vi "SP Align N Complex Waveforms (Linear Interpolation).vi"(4 "Interpolation":bool=TRUE, 5 "Exported Interval":enum16{"Common", "Global"}(ring), 7 "Open Interval? (T)":bool=TRUE, 8 "error in (no error)":errorcluster, 11 "Waveforms In":waveform(cdb)[](array[waveform])) -> (0 "error out":errorcluster, 3 "Aligned Waveforms In":waveform(cdb)[](array[waveform]))   [LabVIEW 2011]
panel:
  in  "Waveform":waveform(cdb)
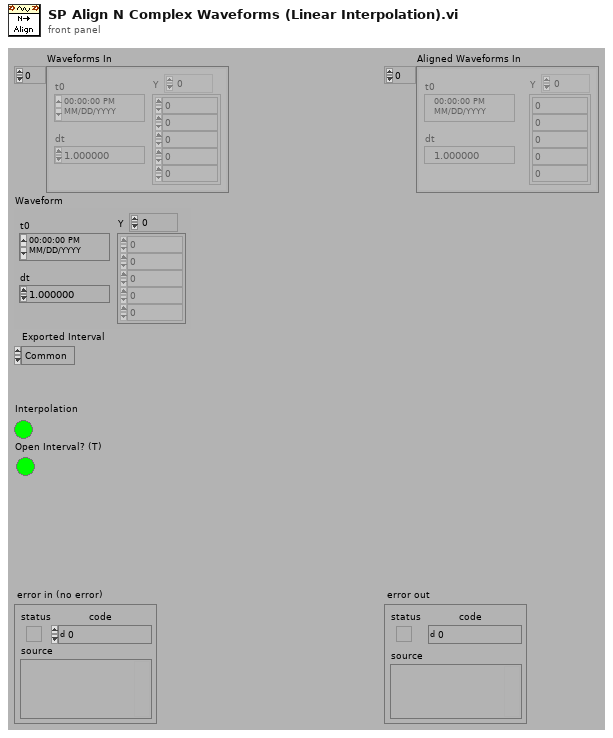
[diagram p1: front panel]
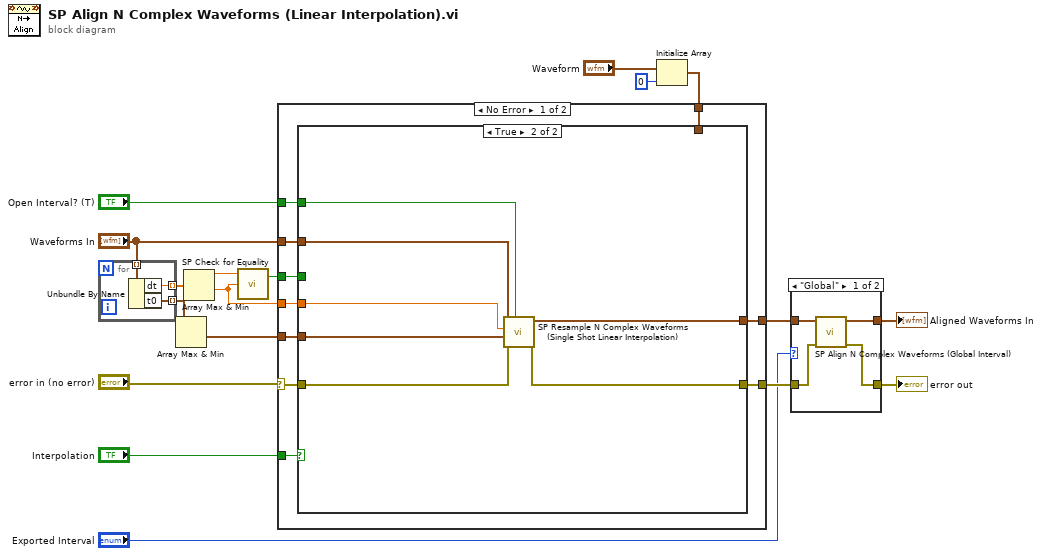
[diagram p0: block diagram]
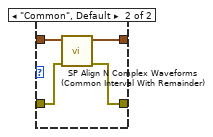
[diagram p2: hidden frame]
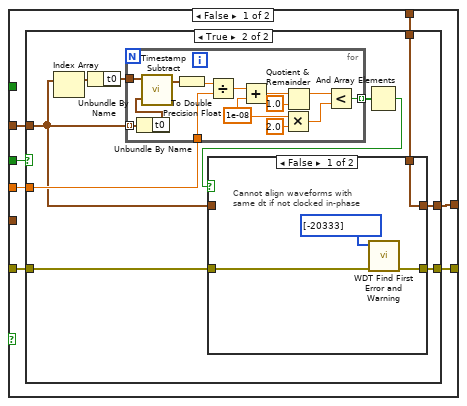
[diagram p3: hidden frame]
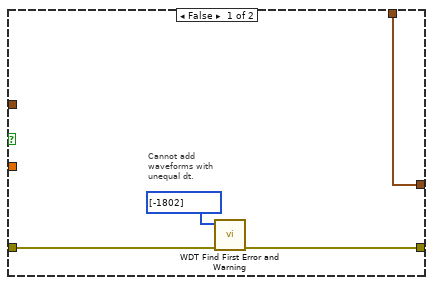
[diagram p4: hidden frame]
diagram:
  n1 = for {
    tunnel: "Waveforms In" -> [w21] mode=indexing
    tunnel: [w20] -> w18 mode=indexing
    tunnel: [w19] -> w2 mode=indexing
    n2 = Unbundle By Name(w21) -> ("dt"=w20:dbl, "t0"=w19:timestamp)
  }
  n3 = Array Max & Min(array=w2) -> (min value=w1:timestamp)  [unwired: 3 out]
  n4 = Array Max & Min(array=w18) -> (max value=w5:dbl, min value=w4:dbl)  [unwired: 2 out]
  n5 = call "SP Check for Equality.vi"("n2"=w4, "n1"=w5) -> ("equal?"=w3:bool)  [unwired: 1 in, 1 out]
  n6 = Initialize Array("Waveform", 0 ("dimension size")) -> (w7:waveform(cdb)[])
  n7 = case shown="No Error" "error in (no error)" {
    selector: "error in (no error)" -> [w30 w81]
    tunnel: [w29 w81] -> w14
    tunnel: w7 -> [w31 w80]
    tunnel: [w28 w80] -> w15
    tunnel: "Interpolation" -> [w27 _]
    tunnel: "Open Interval? (T)" -> [w26 _]
    tunnel: w4 -> [w25 _]
    tunnel: "Waveforms In" -> [w24 _]
    tunnel: w3 -> [w23 _]
    tunnel: w1 -> [w22 _]
    frame No Error {
      n8 = case shown="True" w27 {
        tunnel: w31 -> [w38 _]
        tunnel: w30 -> [w37 w78]
        tunnel: [w36 w79] -> w29
        tunnel: [w35 w74] -> w28
        tunnel: w26 -> [_ w77]
        tunnel: w25 -> [w33 w76]
        tunnel: w24 -> [w32 w75]
        tunnel: w23 -> [w34 _]
        tunnel: w22 -> [_ w73]
        frame False {
          n9 = case shown="True" w34 {
            tunnel: w38 -> [w39 w50]
            tunnel: w37 -> [w42 w52]
            tunnel: [w41 w51] -> w36
            tunnel: [w39 w49] -> w35
            tunnel: w33 -> [_ w48]
            tunnel: w32 -> [_ w44]
            frame False {
              # "Cannot add\nwaveforms with\nunequal dt."
              n10 = call <vilib>:"WDT Find First Error and Warning.vi"("error in (no error)"=w42, "Error Codes"=i32[] [-1802]) -> ("error out"=w41:errorcluster)  [unwired: 1 in, 4 out]
            }
            frame True {
              n11 = Index Array(array=w44) -> (element=w47:waveform(cdb))  [unwired: 1 in]
              n12 = Unbundle By Name(w47) -> ("t0"=w43:timestamp)
              n13 = for {
                tunnel: w43 -> [w56]
                tunnel: w48 -> [w60]
                tunnel: [w64] -> w46 mode=indexing
                tunnel: w44 -> [w59] mode=indexing
                w57 = 1e-08
                n14 = Unbundle By Name(w59) -> ("t0"=w55:timestamp)
                n15 = call <vilib>:"Timestamp Subtract.vi"("y"=w55, "x"=w56) -> ("x - y"=w54:timestamp)
                n16 = To Double Precision Float(number=w54) -> (double precision float=w53:dbl)
                n17 = Divide(x=w53, y=w60) -> (x/y=w58:dbl)
                n18 = Add(x=w58, y=w57) -> (x+y=w63:dbl)
                n19 = Multiply(x=w57, y=2.0) -> (x*y=w61:dbl)
                n20 = Quotient & Remainder(x=w63, y=1.0) -> (x-y*floor(x/y)=w65:dbl)  [unwired: 1 out]
                n21 = Less?(x=w65, y=w61) -> (x < y?=w64:bool)
              }
              n22 = And Array Elements(Boolean array=w46) -> (logical AND=w45:bool)
              n23 = case shown="False" w45 {
                tunnel: [w68 w71] -> w51
                tunnel: w52 -> [w67 w71]
                tunnel: w50 -> [w70 _]
                tunnel: w44 -> [_ w72]
                tunnel: [w70 w72] -> w49
                frame False {
                  # "Cannot align waveforms with\nsame dt if not clocked in-phase"
                  n24 = call <vilib>:"WDT Find First Error and Warning.vi"("error in (no error)"=w67, "Error Codes"=i32[] [-20333]) -> ("error out"=w68:errorcluster)  [unwired: 1 in, 4 out]
                }
                frame True {
                }
              }
            }
          }
        }
        frame True {
          n25 = call "SP Resample N Complex Waveforms (Single Shot Linear Interpolation).vi"("open interval? (T)"=w77, "error in (no error)"=w78, "t0"=w73, "dt"=w76, "waveforms in"=w75) -> ("error out"=w79:errorcluster, "resampled waveforms out"=w74:waveform(cdb)[])  [unwired: 5 out]
        }
      }
    }
    frame Error {
      # "An empty waveform is \nwritten out"
      # "Incoming Error"
    }
  }
  n26 = case shown="\"Global\"" "Exported Interval" {
    tunnel: w15 -> [w83 w86]
    tunnel: [w85 w89] -> w13
    tunnel: w14 -> [w84 w88]
    tunnel: [w82 w87] -> w6
    frame "Global" {
      n27 = call "SP Align N Complex Waveforms (Global Interval).vi"("error in"=w84, "waveforms in"=w83) -> ("error out"=w85:errorcluster, "waveforms out"=w82:waveform(cdb)[])  [unwired: 1 in, 7 out]
    }
    frame "Common", Default {
      n28 = call "SP Align N Complex Waveforms (Common Interval With Remainder).vi"("error in"=w88, "waveforms in"=w86) -> ("error out"=w89:errorcluster, "intersecting waveforms out"=w87:waveform(cdb)[])  [unwired: 8 out]
    }
  }
  "error out" <- w13
  "Aligned Waveforms In" <- w6
